vi "control_var_gen.vi"(2 "keys pressed":T3(array[ring])) -> (6 "out_panel":T2, 7 "out_error":T1)   [LabVIEW 2012]
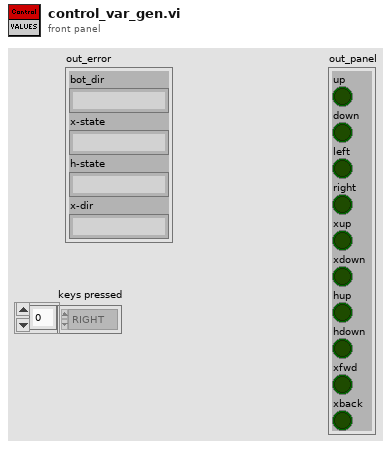
[diagram p1: front panel]
types:
  T1 = cluster{"bot_dir":string, "x-state":string, "h-state":string, "x-dir":string}
  T2 = cluster{"up":bool, "down":bool, "left":bool, "right":bool, "xup":bool, "xdown":bool, "hup":bool, "hdown":bool, "xfwd":bool, "xback":bool}
  T3 = enum16{"0", "1", "2", "3", "4", "5", "6", "7", "8", "9", "A", "B", "C", "D", "E", "F", "G", "H", "I", "J", "K", "L", "M", "N", "O", "P", "Q", "R", "S", "T", "U", "V", "W", "X", "Y", "Z", "F1", "F2", "F3", "F4", "F5", "F6", "F7", "F8", "F9", "F10", "F11", "F12", "F13", "F14", "F15", "ADD", "BACK", "BACKSLASH", "CAPITAL", "COMMA", "DECIMAL", "DELETE", "DIVIDE", "DOWN", "END", "EQUALS", "ESCAPE", "GRAVE (`)", "HOME", "INSERT", "LBRACKET", "LCONTROL", "LEFT", "L ALT", "LSHIFT", "LWIN", "MINUS", "MULTIPLY", "NEXT", "NUMLOCK", "NUMPAD_0", "NUMPAD_1", "NUMPAD_2", "NUMPAD_3", "NUMPAD_4", "NUMPAD_5", "NUMPAD_6", "NUMPAD_7", "NUMPAD_8", "NUMPAD_9", "PAUSE", "PERIOD", "PRIOR (PG UP)", "RBRACKET", "RCONTROL", "RETURN", "RIGHT", "R ALT", "RSHIFT", "RWIN", "SCROLL", "SEMICOLON", "SLASH", "SPACE", "SUBTRACT", "TAB", "UP", "ENTER (num pad)", "' (quote)"}[]
  T4 = enum16{"0", "1", "2", "3", "4", "5", "6", "7", "8", "9", "A", "B", "C", "D", "E", "F", "G", "H", "I", "J", "K", "L", "M", "N", "O", "P", "Q", "R", "S", "T", "U", "V", "W", "X", "Y", "Z", "F1", "F2", "F3", "F4", "F5", "F6", "F7", "F8", "F9", "F10", "F11", "F12", "F13", "F14", "F15", "ADD", "BACK", "BACKSLASH", "CAPITAL", "COMMA", "DECIMAL", "DELETE", "DIVIDE", "DOWN", "END", "EQUALS", "ESCAPE", "GRAVE (`)", "HOME", "INSERT", "LBRACKET", "LCONTROL", "LEFT", "L ALT", "LSHIFT", "LWIN", "MINUS", "MULTIPLY", "NEXT", "NUMLOCK", "NUMPAD_0", "NUMPAD_1", "NUMPAD_2", "NUMPAD_3", "NUMPAD_4", "NUMPAD_5", "NUMPAD_6", "NUMPAD_7", "NUMPAD_8", "NUMPAD_9", "PAUSE", "PERIOD", "PRIOR (PG UP)", "RBRACKET", "RCONTROL", "RETURN", "RIGHT", "R ALT", "RSHIFT", "RWIN", "SCROLL", "SEMICOLON", "SLASH", "SPACE", "SUBTRACT", "TAB", "UP", "ENTER (num pad)", "' (quote)"}
  T5 = cluster{"up":bool, "down":bool, "left":bool, "right":bool, "up/fwd":bool, "down/back":bool, "up/fwd":bool, "down/back":bool, "up/fwd":bool, "down/back":bool}
  T6 = cluster{"String":string, "control_val":string, "control_val":string, "control_val":string}
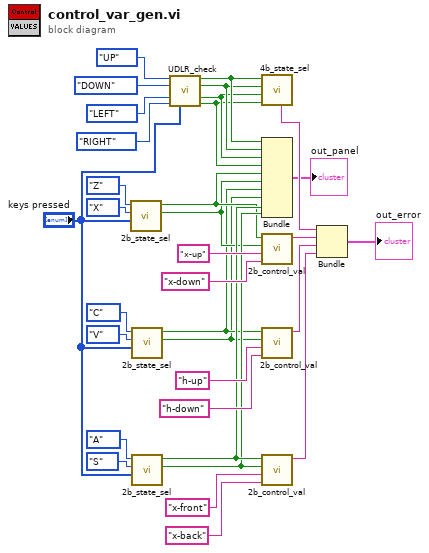
[diagram p0: block diagram]
diagram:
  n1 = call "2b_state_sel.vi"("keys pressed"="keys pressed", "down/back"=T4."X" ("y"), "up/fwd"=T4."Z" ("y")) -> ("down/back"=w6:bool, "up/fwd"=w7:bool)  [unwired: 7 in]
  n2 = call "2b_state_sel.vi"("keys pressed"="keys pressed", "down/back"=T4."V" ("y"), "up/fwd"=T4."C" ("y")) -> ("down/back"=w1:bool, "up/fwd"=w2:bool)  [unwired: 7 in]
  n3 = call "2b_state_sel.vi"("keys pressed"="keys pressed", "down/back"=T4."S" ("y"), "up/fwd"=T4."A" ("y")) -> ("down/back"=w20:bool, "up/fwd"=w21:bool)  [unwired: 7 in]
  n4 = call "UDLR_check.vi"("up"=T4."UP" ("y"), "down"=T4."DOWN" ("y"), "left"=T4."LEFT" ("y"), "right"=T4."RIGHT" ("y"), "keys pressed"="keys pressed") -> ("up"=w14:bool, "down"=w13:bool, "left"=w12:bool, "right"=w11:bool)  [unwired: 7 in]
  n5 = call "4b_state_sel.vi"("Right"=w11, "Left"=w12, "Down"=w13, "Up"=w14) -> ("String"=w19:string)  [unwired: 7 in]
  n6 = Bundle("up"=w14, "down"=w13, "left"=w12, "right"=w11, "up/fwd"=w7, "down/back"=w6, "up/fwd"=w2, "down/back"=w1, "up/fwd"=w21, "down/back"=w20) -> (→"out_panel":T5)  [unwired: 1 in]
  n7 = call "2b_control_val.vi"(8:"down/back"="x-down" ("down/back"), "up/fwd"="x-up", 10:"down/back"=w6, "Up/fwd"=w7) -> ("control_val"=w18:string)  [unwired: 7 in]
  n8 = call "2b_control_val.vi"(8:"down/back"="h-down" ("down/back"), "up/fwd"="h-up", 10:"down/back"=w1, "Up/fwd"=w2) -> ("control_val"=w17:string)  [unwired: 7 in]
  n9 = call "2b_control_val.vi"(8:"down/back"="x-back" ("down/back"), "up/fwd"="x-front", 10:"down/back"=w20, "Up/fwd"=w21) -> ("control_val"=w16:string)  [unwired: 7 in]
  n10 = Bundle("String"=w19, "control_val"=w18, "control_val"=w17, "control_val"=w16) -> (→"out_error":T6)  [unwired: 1 in]
